vi "PropertyChangedEventCallbackForCapturedFrames.vi"(4 "?":refnum<vi>, 5 "Event Data":cluster{"sender":refnum<k24>, "e":refnum<k24>}, 6 "Control Ref":refnum<k24>, 7 "Event Common Data":T1) -> ()   [LabVIEW 2018]
uses:
  C:/Users/Dell/Desktop/SIMImaging/Dependencies/PVCamNET.dll
  Dependencies/PVCamNET.dll
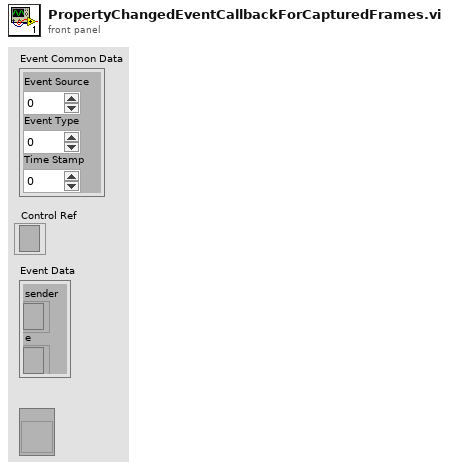
[diagram p1: front panel]
types:
  T1 = cluster{"Event Source":i32, "Event Type":u32, "Time Stamp":u32}
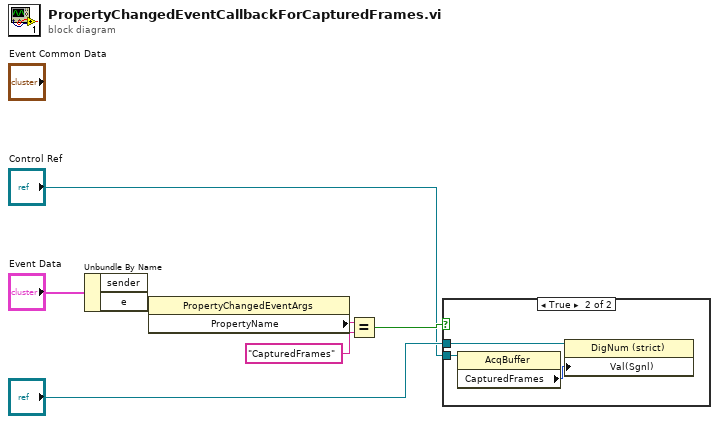
[diagram p0: block diagram]
diagram:
  n1 = Unbundle By Name("Event Data") -> ("e"=w6:refnum<k24>)  [unwired: 1 out]
  n2 = property class="PropertyChangedEventArgs"(reference=w6) -> ("PropertyName"=w5:string)  [unwired: 1 in, 2 out]
  n3 = Equal?(x=w5, y="CapturedFrames") -> (x = y?=w3:bool)
  n4 = case shown="True" w3 {
    tunnel: "?" -> [_ w10]
    tunnel: "Control Ref" -> [_ w9]
    frame False {
    }
    frame True {
      n5 = property class="AcqBuffer"(reference=w9) -> ("CapturedFrames"=w8:i32)  [unwired: 1 in, 2 out]
      n6 = property class="DigNum (strict)"(reference=w10, "Val(Sgnl)"=w8) -> ()  [unwired: 1 in, 2 out]
    }
  }
